vi "DVS_LabVIEWController_april2015.vi"() -> ()   [LabVIEW 2014]
doc: "This example demonstrates temperature control and monitoring.\n\nNote:\nBefore start this VI is it necessary:\n\n- preconfigure some specific parameters that are not supported by this driver (e.g. PV-I/O Type, Linearization type, Alarm Input Values... ) by Quick Codes, or by Eurotherm iTools or by instrument front panel controls\n- enter correct VISA Resource Descriptor, Device Address and Baud Rate into front-panel controls"
uses:
  <vilib>/Instr/_visa.llb/VISA Configure Serial Port (Instr).vi
  Environmental Chamber LabVIEW and Instruments/Drivers and Software/keithley_6430/Keithley 6430/Public/Data/Read (Single Point).vi
  Environmental Chamber LabVIEW and Instruments/Drivers and Software/LabVIEW 8.2 Drivers/keithley_24xx/Keithley 24XX/Public/Data/Read (Single Point).vi
  <vilib>/Utility/file.llb/Write To Spreadsheet File (string).vi
  Environmental Chamber LabVIEW and Instruments/Drivers and Software/keithley_24xx/Keithley 24XX/Keithley 24XX.lvlib
  Environmental Chamber LabVIEW and Instruments/Drivers and Software/keithley_6430/Keithley 6430/Keithley 6430.lvlib
panel:
  out "F_o (MHz)":dbl
  out "Waveform Chart 8":cluster{dbl}(graph)
  out "Waveform Chart 9":cluster{"Measurement":dbl}(graph)
  out "Waveform Chart 4":cluster{"Resistance":sgl}(graph)
  in  "Keithley 6430":bool
  in  "Keithley 2422":bool
  in  "Keithley 2423":bool
  in  "Keithley 2421":bool
  in  "stop":bool
  in  "Keithley 2420":bool
  in  "J-KEM":bool
  out "Start Time":string
  out "Elapsed (min)":dbl caption="Elapsed Time (s)"
  out "Data\nfile\npath":path
  in  "Comments":string
  out "Program Errors":errorcluster
  in  "Delay between data points (s)":dbl min=0.0 max=30.0 format="%#_13g"
  in  "Stop after (min)":dbl
  in  "Auto stop?":bool
  out "Ohm":dbl format="%.4e"
  out "MHz":dbl format="%.6f"
  out "Waveform Chart 7":cluster{dbl, "Resistance out":dbl}(graph)
  out "Waveform Chart 5":cluster{dbl}(graph)
  in  "Clear all charts":bool
  out "Waveform Chart 6":cluster{dbl}(graph)
  out "O2 Concentration (PPM)":dbl
  out "Waveform Chart":cluster{dbl}(graph)
  out "Torr":dbl
  out "%":dbl
  out "atm":dbl
  in  "Com Port":i32(ring) items=["Com 1", "Com 2", "Com 3", "Com 4", "Com 5", "Com 6", "COM 7", "COM 8", "COM 9", "COM 10", "COM 11", "COM 12", "com 13", "COM 14"]
  in  "Baud Rate 2":i32(ring)=2 items=["2400", "4800", "9600", "19200", "38400", "57600", "115200"]
  in  "Com Port 2":i32(ring) items=["Com 1", "Com 2", "Com 3", "Com 4", "Com 5", "Com 6", "COM 7", "COM 8", "COM 9", "COM 10", "COM 11", "COM 12", "com 13", "COM 14"]
  # "Configuring Instrument\n \nPlease Wait......\n\nChart will update in 20 sec"
  # "O2 Partial Pressure"
  # "SetNag\nO2 Pump"
  # "Rapidox O2 Sensor"
  # "°C"
  # "Sample Temperature"
  # "Mass adsorbed (g)"
  # "Keithley 6430 Resistance"
  # "Ohm"
  # "Keithley 2420 Resistance"
  # "Ohm"
  # "Setup"
  # "Instruments Connected:"
  # "Timing"
  # "SRS QCM"
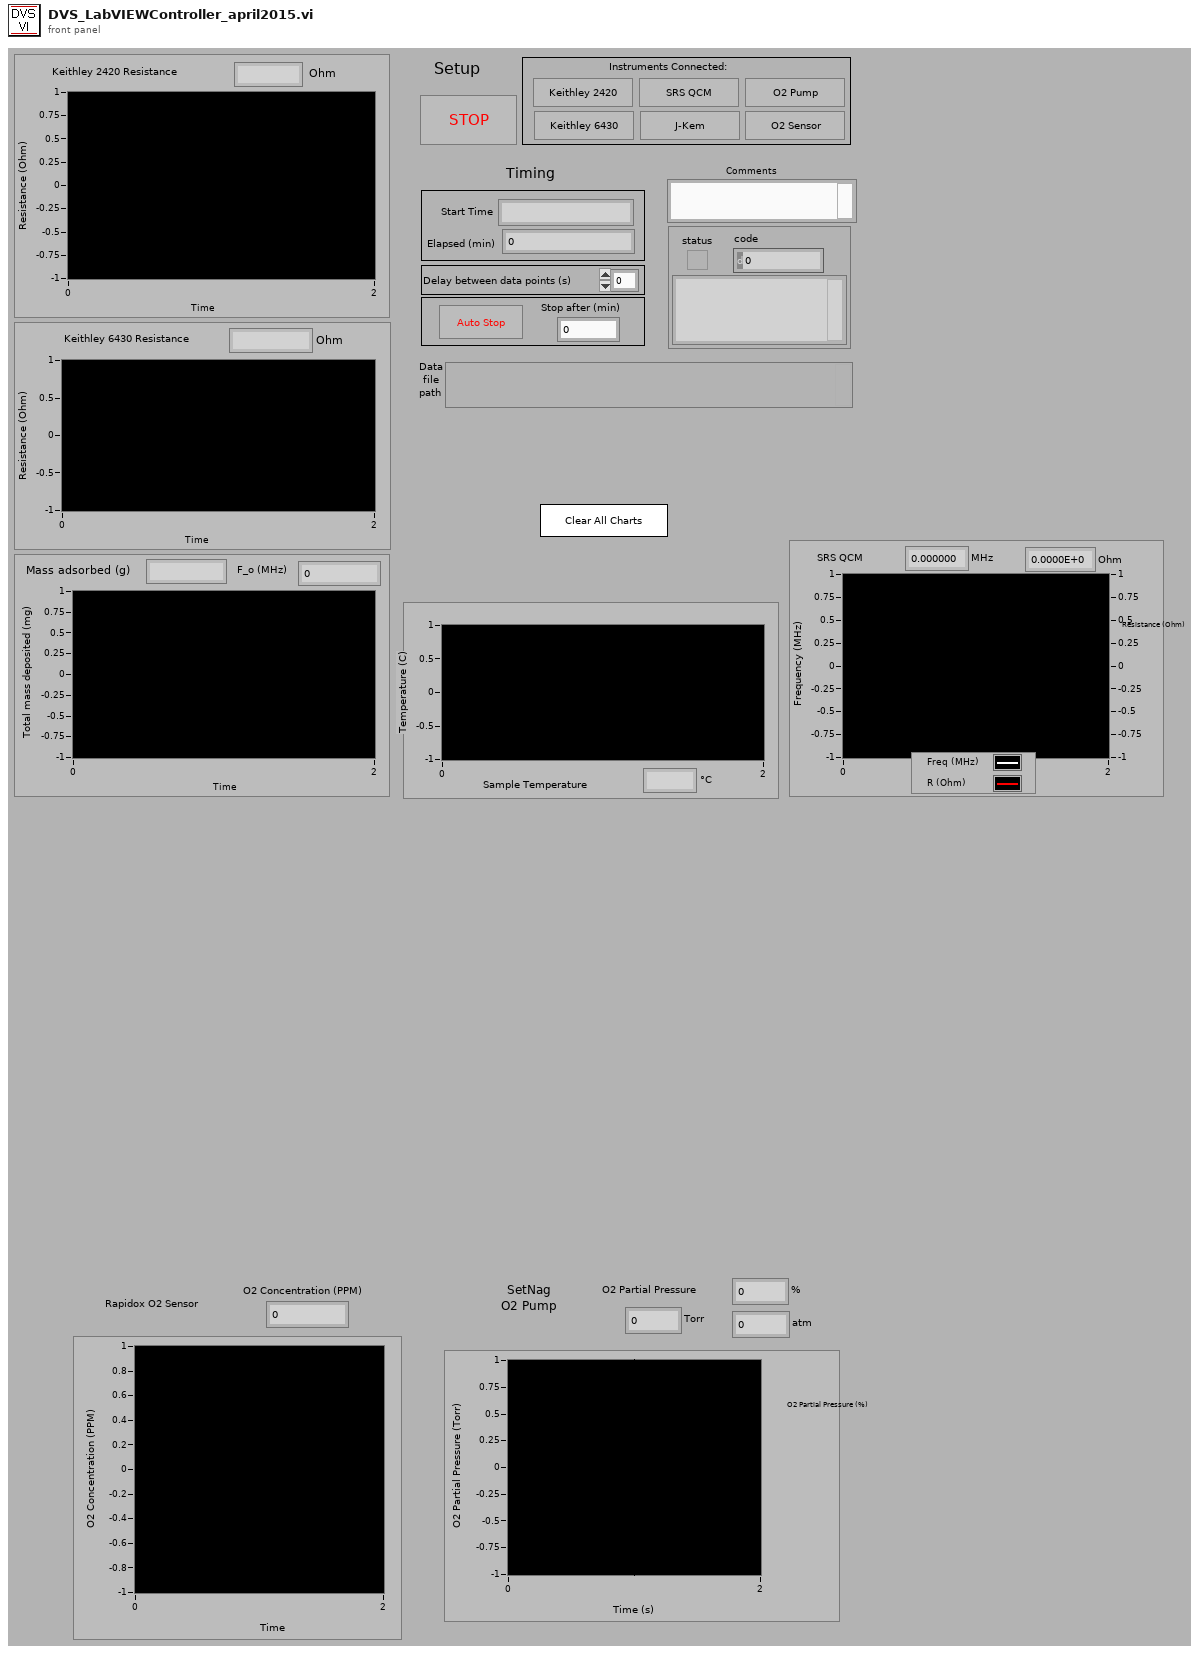
[diagram p1: front panel]
types:
  T1 = enum16{"open", "open or create", "create or replace", "create", "open (read only)"}
  T2 = enum16{"no parity", "odd parity", "even parity", "mark parity", "space parity"}
  T3 = cluster{bool, "VISA resource name":refnum<visa-resource-name>, "error out":errorcluster}
  T4 = cluster{bool, "VISA resource name out":refnum<visa-resource-name>, "error out":errorcluster}
  T5 = cluster{bool, "VISA out":refnum<visa-resource-name>, "error out":errorcluster}
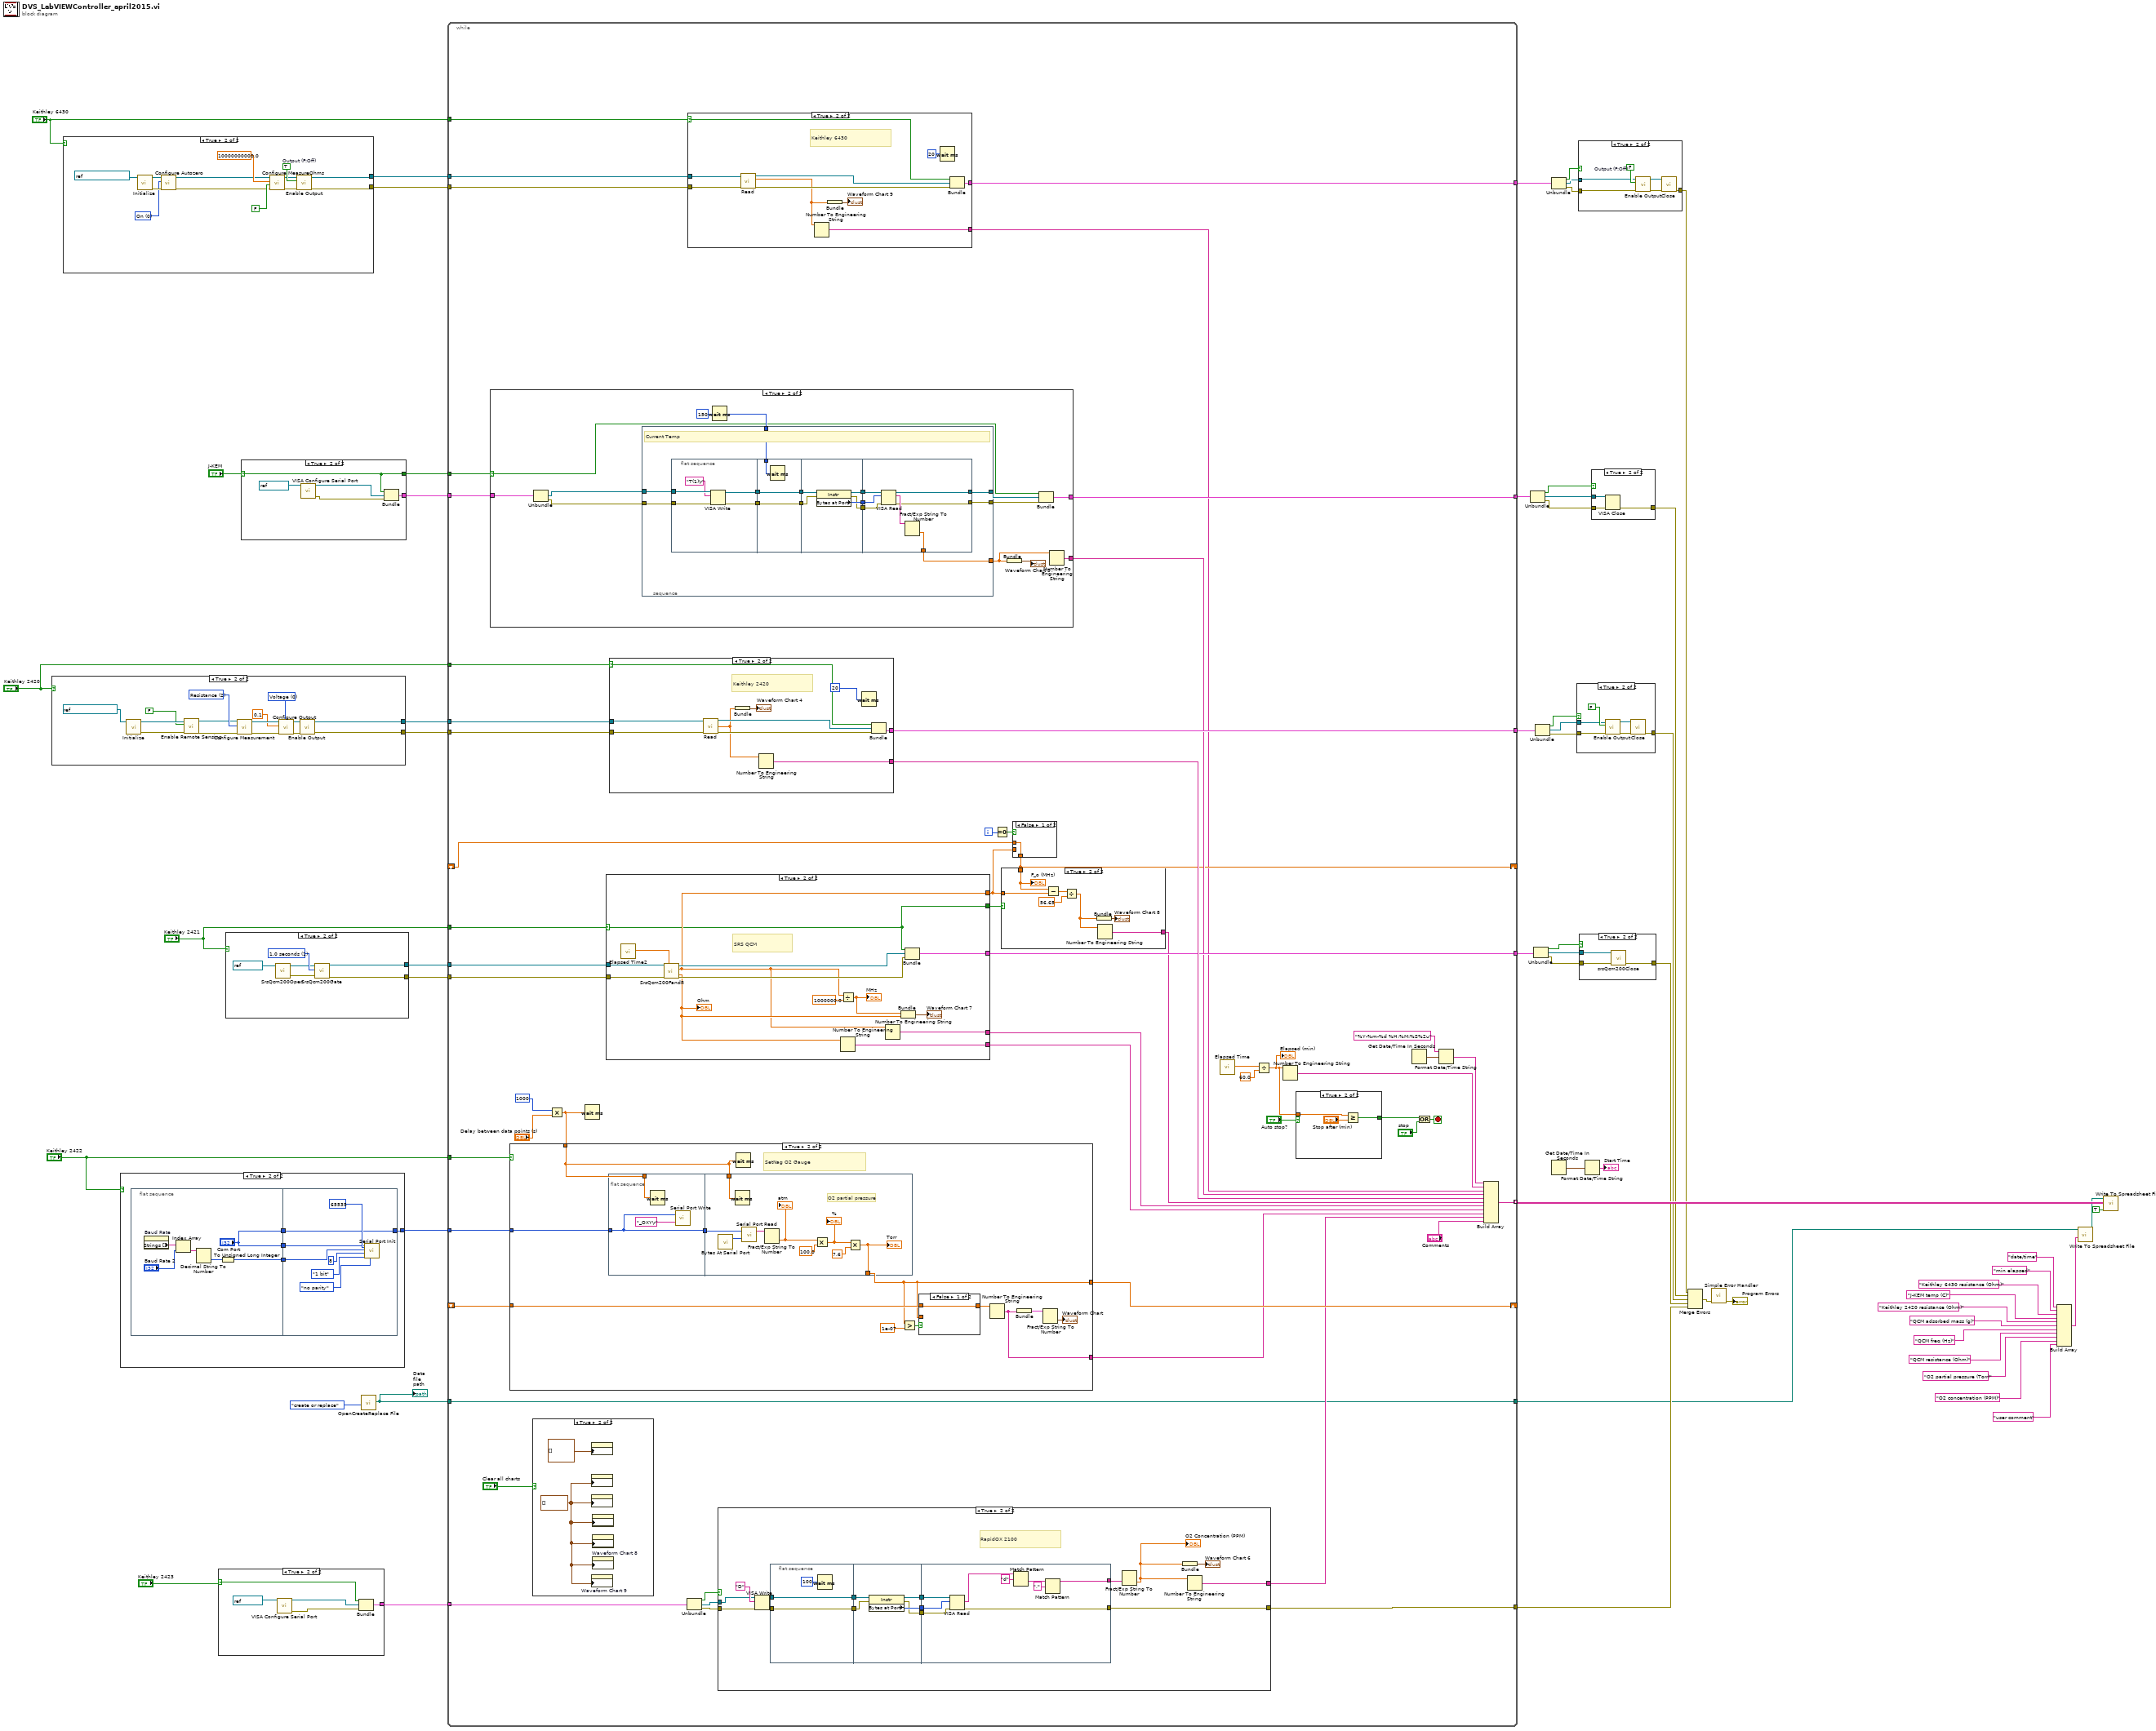
[diagram p0: block diagram]
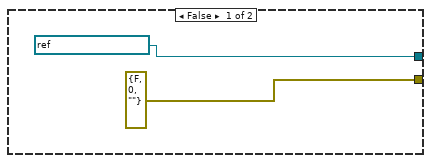
[diagram p3: hidden frame]
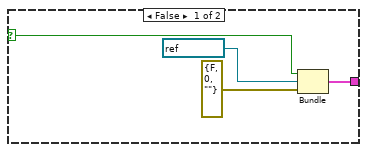
[diagram p4: hidden frame]
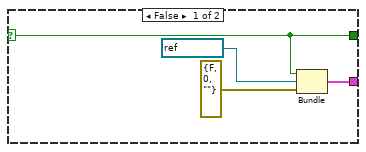
[diagram p6: hidden frame]
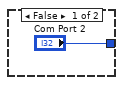
[diagram p7: hidden frame]
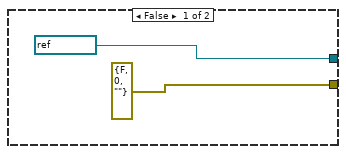
[diagram p9: hidden frame]
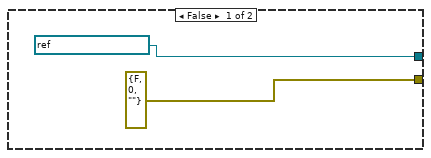
[diagram p11: hidden frame]
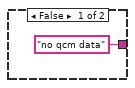
[diagram p12: hidden frame]
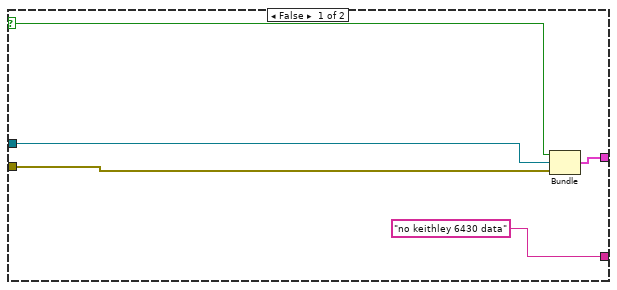
[diagram p13: hidden frame]
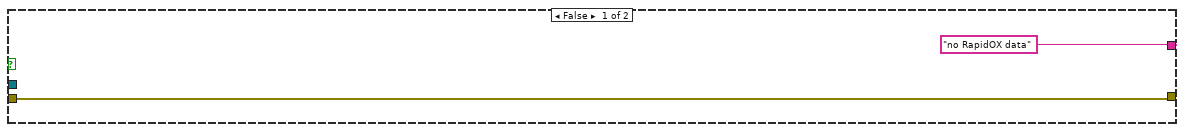
[diagram p16: hidden frame]
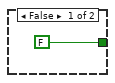
[diagram p17: hidden frame]
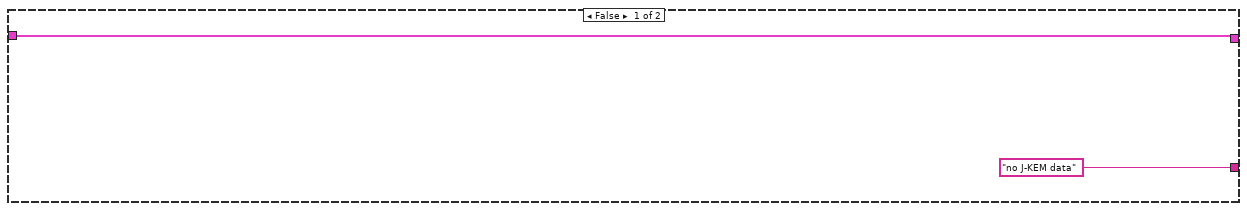
[diagram p18: hidden frame]
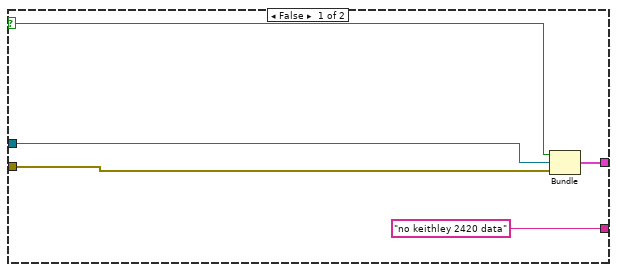
[diagram p19: hidden frame]
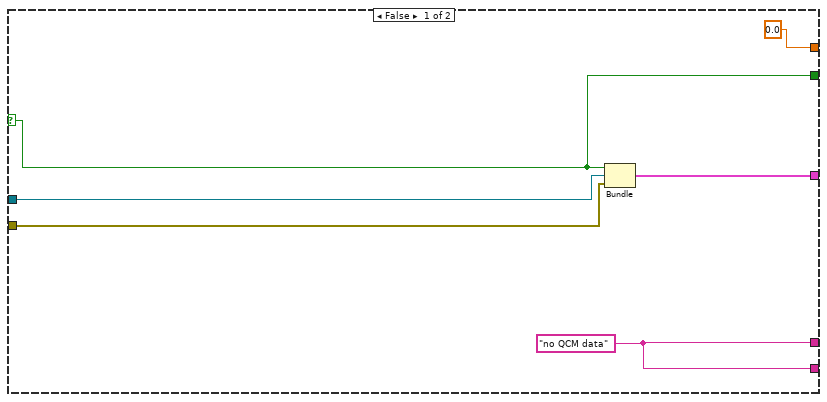
[diagram p20: hidden frame]
diagram:
  n1 = case shown="True" "Keithley 2420" {
    tunnel: [refnum<visa-resource-name> "GPIB1::24::INSTR" ("VISA resource name") w68] -> w54
    tunnel: [errorcluster {"status"=FALSE, "code"=0, "source"=""} ("error out") w63] -> w53
    frame False {
    }
    frame True {
      w70 = u16 0 items=["Voltage", "Current"] ("Source Mode  (0: Voltage)")
      w75 = u16 2 items=["Volts", "Current", "Resistance"] ("Function (0: Volts)")
      n2 = call "Initialize.vi"("VISA resource name"=refnum<visa-resource-name> "GPIB1::24::INSTR") -> ("error out"=w64:errorcluster, "VISA resource name out"=w67:refnum<visa-resource-name>)  [unwired: 9 in]
      n3 = call "Enable Remote Sensing.vi"("error in (no error)"=w64, "Enable Remote Sensing (T: Enable)"=FALSE ("4-wire?"), "VISA resource name"=w67) -> ("error out"=w65:errorcluster, "VISA resource name out"=w66:refnum<visa-resource-name>)  [unwired: 7 in]
      n4 = call "Configure Measurement.vi"("error in (no error)"=w65, "Function (0: Volts)"=w75, "VISA resource name"=w66) -> ("error out"=w74:errorcluster, "VISA resource name out"=w73:refnum<visa-resource-name>)  [unwired: 7 in]
      n5 = call "Configure Output.vi"("Source Mode  (0: Voltage)"=w70, "error in (no error)"=w74, "Output Level (0)"=0.1 ("Applied Voltage (V)"), "VISA resource name"=w73) -> ("error out"=w72:errorcluster, "VISA resource name out"=w71:refnum<visa-resource-name>)  [unwired: 6 in]
      n6 = call "Enable Output.vi"("error in (no error)"=w72, "VISA resource name"=w71) -> ("error out"=w63:errorcluster, "VISA resource name out"=w68:refnum<visa-resource-name>)  [unwired: 8 in]
    }
  }
  n7 = case shown="True" "Keithley 6430" {
    tunnel: [refnum<visa-resource-name> "GPIB0::29::INSTR" ("VISA resource name") w86] -> w6
    tunnel: [errorcluster {"status"=FALSE, "code"=0, "source"=""} ("error out") w87] -> w5
    frame False {
    }
    frame True {
      w82 = u16 0 items=["On", "Off", "Once"] ("Autozero  (0: On)")
      w90 = TRUE  # Output (F:Off)
      n8 = call "Initialize.vi"("VISA resource name"=refnum<visa-resource-name> "GPIB0::29::INSTR") -> ("error out"=w83:errorcluster, "VISA resource name out"=w84:refnum<visa-resource-name>)  [unwired: 4 in, 5 out]
      n9 = call "Configure Autozero.vi"("error in (no error)"=w83, "Autozero  (0: On)"=w82, "VISA resource name"=w84) -> ("error out"=w79:errorcluster, "VISA resource name out"=w80:refnum<visa-resource-name>)  [unwired: 7 in]
      n10 = call "Configure MeasureOhms.vi"("error in (no error)"=w79, "Auto Range (T:Enable)"=FALSE, "Resistance Range [Ohms]"=10000000000.0, "VISA resource name"=w80) -> ("error out"=w91:errorcluster, "VISA resource name out"=w89:refnum<visa-resource-name>)  [unwired: 2 in, 4 out]
      n11 = call "Enable Output.vi"("error in (no error)"=w91, "Enable Output (F:Off)"=w90, "VISA resource name"=w89) -> ("error out"=w87:errorcluster, "VISA resource name out"=w86:refnum<visa-resource-name>)  [unwired: 7 out]
    }
  }
  n12 = case shown="True" "Keithley 2422" {
    tunnel: ["Com Port 2" w93] -> w50
    frame False {
    }
    frame True {
      n13 = flat-sequence {
        tunnel: ["Com Port"] -> w96
        tunnel: [w98] -> w95
        tunnel: ["Com Port"] -> w94
        tunnel: w96 -> [w104]
        tunnel: w95 -> [w103]
        tunnel: w94 -> [w105]
        tunnel: [w105] -> w93
        frame #0 {
          n14 = property on="Baud Rate" class="Ring (strict)"() -> ("Strings []"=w100:string[])  [unwired: 2 in, 2 out]
          n15 = Index Array(array=w100, index="Baud Rate 2") -> (element=w101:string)
          n16 = Decimal String To Number(string=w101) -> (number=w99:i32)  [unwired: 2 in, 1 out]
          n17 = To Unsigned Long Integer(number=w99) -> (unsigned 32bit integer=w98:u32)
        }
        frame #1 {
          n18 = call <vilib>:"Serial Port Init.vi"("parity"=T2."no parity", "buffer size"=u16 65535, "stop bits"=enum16{"1 bit", "1.5 bits", "2 bits"}."1 bit", "data bits"=u16 8, "baud rate"=w103, "port number"=w104) -> ()  [unwired: 1 in, 1 out]
        }
      }
    }
  }
  n19 = case shown="True" "Keithley 2423" {
    selector: "Keithley 2423" -> [w110 w115]
    tunnel: [w111 w116] -> w19
    frame False {
      n20 = Bundle(w110, "VISA resource name"=refnum<visa-resource-name> "COM7", "error out"=errorcluster {"status"=FALSE, "code"=0, "source"=""}) -> (w111:T3)  [unwired: 1 in]
    }
    frame True {
      n21 = call-poly "VISA Configure Serial Port"("VISA resource name"=refnum<visa-resource-name> "COM7") -> ("VISA resource name out"=w117:refnum<visa-resource-name>, "error out"=w114:errorcluster)  [unwired: 13 in]
      n22 = Bundle(w115, "VISA resource name out"=w117, "error out"=w114) -> (w116:T4)  [unwired: 1 in]
    }
  }
  n23 = case shown="True" "Keithley 2421" {
    tunnel: [refnum<visa-resource-name> "COM6" ("VISA in") w122] -> w52
    tunnel: [errorcluster {"status"=FALSE, "code"=0, "source"=""} ("error out") w121] -> w51
    frame False {
    }
    frame True {
      w126 = u16 1 items=["0.1 seconds", "1.0 seconds", "10.0 seconds"] ("Gate in")
      n24 = call "SrsQcm200Open.vi"("VISA in"=refnum<visa-resource-name> "COM6") -> ("error out"=w123:errorcluster, "VISA out"=w124:refnum<visa-resource-name>)  [unwired: 4 in]
      n25 = call "SrsQcm200Gate.vi"("VISA in"=w124, "Gate in"=w126, "error in (no error)"=w123) -> ("VISA out"=w122:refnum<visa-resource-name>, "error out"=w121:errorcluster)  [unwired: 14 in, 1 out]
    }
  }
  n26 = case shown="True" "J-KEM" {
    selector: "J-KEM" -> [w127 w132]
    tunnel: [w128 w133] -> w39
    tunnel: [w127 w132] -> w32
    frame False {
      n27 = Bundle(w127, "VISA resource name"=refnum<visa-resource-name> "COM3", "error out"=errorcluster {"status"=FALSE, "code"=0, "source"=""}) -> (w128:T3)  [unwired: 1 in]
    }
    frame True {
      n28 = call-poly "VISA Configure Serial Port"("VISA resource name"=refnum<visa-resource-name> "COM3") -> ("VISA resource name out"=w134:refnum<visa-resource-name>, "error out"=w131:errorcluster)  [unwired: 13 in]
      n29 = Bundle(w132, "VISA resource name out"=w134, "error out"=w131) -> (w133:T4)  [unwired: 1 in]
    }
  }
  n30 = call "OpenCreateReplace File.vi"("function (open:0)"=T1."create or replace") -> ("new file path"=w15:path)  [unwired: 7 in, 3 out]
  "Data\nfile\npath" <- w15
  n31 = while {
    shift-right: [w189] -> _
    shift-left: _ -> [w188]
    tunnel: [w186] -> w56 mode=indexing
    tunnel: "Keithley 2420" -> [w152]
    tunnel: w54 -> [w184]
    tunnel: w53 -> [w183]
    tunnel: w52 -> [w182]
    tunnel: w51 -> [w181]
    tunnel: "Keithley 2421" -> [w179]
    tunnel: "Keithley 2422" -> [w172]
    tunnel: w50 -> [w178]
    tunnel: [w174] -> w47
    tunnel: [w173] -> w43
    tunnel: w39 -> [w171]
    tunnel: [w170] -> w37
    tunnel: w32 -> [w168]
    tunnel: w19 -> [w161]
    tunnel: [w156] -> w17
    tunnel: [w151] -> w16
    tunnel: w15 -> [w151]
    shift-right: [w145] -> _
    shift-left: _ -> [w144]
    tunnel: w6 -> [w143]
    tunnel: w5 -> [w142]
    tunnel: [w141] -> w3
    tunnel: "Keithley 6430" -> [w140]
    i -> [w137]
    stop <- w166 stop-if-true
    n32 = case shown="True" w168 {
      selector: w168 -> [_ w260]
      tunnel: w171 -> [w258 w265]
      tunnel: [w258 w263] -> w170
      tunnel: ["no J-KEM data" w261] -> w169
      frame False {
      }
      frame True {
        w269 = u32 150 ("milliseconds to wait")
        n33 = Unbundle(w265) -> ("VISA resource name out"=w264:refnum<visa-resource-name>, "error out"=w259:errorcluster)  [unwired: 1 out]
        n34 = stacked-sequence {
          tunnel: w264 -> [w275]
          tunnel: w259 -> [w274]
          tunnel: w269 -> [w273]
          tunnel: [w271] -> w266
          tunnel: [w270] -> w267
          tunnel: [w272] -> w262
          frame #0 {
            # "Current Temp"
            n35 = flat-sequence {
              tunnel: w275 -> [w287]
              tunnel: w274 -> [w286]
              tunnel: [w284] -> w282
              tunnel: [w283] -> w281
              tunnel: w273 -> [w290]
              tunnel: [w289] -> w280
              tunnel: w282 -> [w289]
              tunnel: w281 -> [w288]
              tunnel: [w288] -> w279
              tunnel: w280 -> [w295]
              tunnel: w279 -> [w294]
              tunnel: [w293] -> w278
              tunnel: [w292] -> w277
              tunnel: [w291] -> w276
              tunnel: w278 -> [w302]
              tunnel: w277 -> [w301]
              tunnel: w276 -> [w300]
              tunnel: [w297] -> w270
              tunnel: [w298] -> w271
              tunnel: [w296] -> w272
              frame #0 {
                n36 = VISA Write(VISA resource name=w287, write buffer="T(1)\r", error in (no error)=w286) -> (VISA resource name out=w284:refnum<visa-resource-name>, error out=w283:errorcluster)  [unwired: 1 out]
              }
              frame #1 {
                n37 = Wait (ms)(milliseconds to wait=w290) -> ()  [unwired: 1 out]
              }
              frame #2 {
                n38 = property class="Instr"(reference=w295, error in=w294) -> (reference out=w293:refnum<visa-resource-name>, error out=w291:errorcluster, "Bytes at Port"=w292:u32)
              }
              frame #3 {
                n39 = VISA Read(VISA resource name=w302, byte count=w301, error in (no error)=w300) -> (VISA resource name out=w298:refnum<visa-resource-name>, read buffer=w299:string, error out=w297:errorcluster)  [unwired: 1 out]
                n40 = Fract/Exp String To Number(string=w299) -> (number=w296:dbl)  [unwired: 3 in, 1 out]
              }
            }
          }
        }
        n41 = Wait (ms)(milliseconds to wait=w269) -> ()  [unwired: 1 out]
        n42 = Bundle(w262) -> (→"Waveform Chart 5":cluster{dbl})  [unwired: 1 in]
        n43 = Bundle(w260, "VISA resource name out"=w266, "error out"=w267) -> (w263:T4)  [unwired: 1 in]
        n44 = Number To Engineering String(4:w262) -> (0:w261:string)  [unwired: 3 in]
      }
    }
    n45 = case shown="True" "Clear all charts" {
      frame False {
      }
      frame True {
        w217 = cluster{dbl}[] [] ("History Data")
        n46 = property on="Waveform Chart 7" class="WFChart (strict)"("History Data"=cluster{dbl, "Resistance out":dbl}[] []) -> ()  [unwired: 2 in, 2 out]
        n47 = property on="Waveform Chart 4" class="WFChart (strict)"("History Data"=w217) -> ()  [unwired: 2 in, 2 out]
        n48 = property on="Waveform Chart 5" class="WFChart (strict)"("History Data"=w217) -> ()  [unwired: 2 in, 2 out]
        n49 = property on="Waveform Chart 9" class="WFChart (strict)"("History Data"=w217) -> ()  [unwired: 2 in, 2 out]
        n50 = property on="Waveform Chart" class="WFChart (strict)"("History Data"=w217) -> ()  [unwired: 2 in, 2 out]
        n51 = property on="Waveform Chart 6" class="WFChart (strict)"("History Data"=w217) -> ()  [unwired: 2 in, 2 out]
        n52 = property on="Waveform Chart 8" class="WFChart (strict)"("History Data"=w217) -> ()  [unwired: 2 in, 2 out]
      }
    }
    n53 = Multiply(x=u32 1000, y="Delay between data points (s)") -> (x*y=w155:dbl)
    n54 = case shown="True" w172 {
      tunnel: [w339 w343] -> w189
      tunnel: w188 -> [w339 w344]
      tunnel: w155 -> [_ w340]
      tunnel: w178 -> [_ w342]
      tunnel: ["no GenAir data" w341] -> w177
      frame False {
      }
      frame True {
        # "SetNag O2 Gauge"
        n55 = flat-sequence {
          tunnel: [w353] -> w350
          tunnel: w340 -> [w355]
          tunnel: w342 -> [w353]
          tunnel: w350 -> [w356]
          tunnel: w340 -> [w363]
          tunnel: [w359] -> w343
          frame #0 {
            n56 = Wait (ms)(milliseconds to wait=w355) -> ()  [unwired: 1 out]
            n57 = call <vilib>:"Serial Port Write.vi"("string to write"="_OXY\r" ("O2 partial press"), "port number"=w353) -> ()  [unwired: 1 out]
          }
          frame #1 {
            # "O2 partial pressure"
            n58 = call <vilib>:"Bytes At Serial Port.vi"() -> ("byte count"=w364:u32)  [unwired: 1 in, 1 out]
            n59 = Wait (ms)(milliseconds to wait=w363) -> ()  [unwired: 1 out]
            n60 = call <vilib>:"Serial Port Read.vi"("requested byte count"=w364, "port number"=w356) -> ("string read"=w362:string)  [unwired: 1 out]
            n61 = Fract/Exp String To Number(string=w362) -> (number=w360:dbl)  [unwired: 3 in, 1 out]
            "atm" <- w360
            n62 = Multiply(x=w360, y=100.0) -> (x*y=w357:dbl)
            "%" <- w357
            n63 = Multiply(x=w357, y=7.6) -> (x*y=w359:dbl)
            "Torr" <- w359
          }
        }
        n64 = Wait (ms)(milliseconds to wait=w340) -> ()  [unwired: 1 out]
        n65 = Greater?(x=w343, y=1e-07) -> (0:w346:bool)
        n66 = case shown="False" w346 {
          tunnel: [w351 w352] -> w345
          tunnel: w343 -> [_ w352]
          tunnel: w344 -> [w351 _]
          frame False {
          }
          frame True {
          }
        }
        n67 = Number To Engineering String(4:w345) -> (0:w341:string)  [unwired: 3 in]
        n68 = Bundle(w341) -> (w348:cluster{string})  [unwired: 1 in]
        n69 = Fract/Exp String To Number(string=w348) -> (number=→"Waveform Chart":cluster{dbl})  [unwired: 3 in, 1 out]
      }
    }
    n70 = Wait (ms)(milliseconds to wait=w155) -> ()  [unwired: 1 out]
    n71 = case shown="True" w179 {
      selector: w179 -> [w318 w324]
      tunnel: w182 -> [w322 w330]
      tunnel: w181 -> [w321 w332]
      tunnel: [w323 w337] -> w180
      tunnel: [w323 w336] -> w176
      tunnel: [w320 w335] -> w173
      tunnel: [0.0 w325] -> w147
      tunnel: [w318 w324] -> w136
      frame False {
        w323 = "no QCM data"
        n72 = Bundle(w318, "VISA out"=w322, "error out"=w321) -> (w320:T5)  [unwired: 1 in]
      }
      frame True {
        # "SRS QCM"
        n73 = call "Elapsed Time2"() -> ("Elapsed Time (s)"=w331:dbl)  [unwired: 12 in, 7 out]
        n74 = call "SrsQcm200FandR.vi"("VISA in"=w330, "Reference time in"=w331, "error in (no error)"=w332) -> ("VISA out"=w328:refnum<visa-resource-name>, "Frequency out"=w325:dbl, "Resistance out"=w327:dbl, "error out"=w329:errorcluster)  [unwired: 6 in, 3 out]
        "Ohm" <- w327
        n75 = Number To Engineering String(4:w327) -> (0:w336:string)  [unwired: 3 in]
        n76 = Divide(x=w325, y=1000000.0) -> (x/y=w326:dbl)
        "MHz" <- w326
        n77 = Number To Engineering String(4:w325) -> (0:w337:string)  [unwired: 3 in]
        n78 = Bundle(w326, "Resistance out"=w327) -> (→"Waveform Chart 7":cluster{dbl, "Resistance out":dbl})  [unwired: 1 in]
        n79 = Bundle(w324, "VISA out"=w328, "error out"=w329) -> (w335:T5)  [unwired: 1 in]
      }
    }
    n80 = case shown="True" w152 {
      selector: w152 -> [w306 w314]
      tunnel: w184 -> [w305 w309]
      tunnel: w183 -> [w304 w308]
      tunnel: [w303 w312] -> w174
      tunnel: ["no keithley 2420 data" w311] -> w175
      frame False {
        n81 = Bundle(w306, "VISA resource name out"=w305, "error out"=w304) -> (w303:T4)  [unwired: 1 in]
      }
      frame True {
        # "Keithley 2420"
        n82 = call-poly "Read.vi"("VISA resource name"=w309, "error in (no error)"=w308) -> ("VISA resource name out"=w315:refnum<visa-resource-name>, "Resistance"=w310:sgl, "error out"=w313:errorcluster)  [unwired: 7 in, 4 out]
        n83 = Bundle("Resistance"=w310) -> (→"Waveform Chart 4":cluster{"Resistance":sgl})  [unwired: 1 in]
        n84 = Number To Engineering String(4:w310) -> (0:w311:string)  [unwired: 3 in]
        n85 = Wait (ms)(milliseconds to wait=u32 20) -> ()  [unwired: 1 out]
        n86 = Bundle(w314, "VISA resource name out"=w315, "error out"=w313) -> (w312:T4)  [unwired: 1 in]
      }
    }
    n87 = Unbundle(w161) -> (w160:bool, "VISA resource name out"=w159:refnum<visa-resource-name>, "error out"=w158:errorcluster)
    n88 = case shown="True" w140 {
      selector: w140 -> [w203 w213]
      tunnel: w143 -> [w202 w210]
      tunnel: w142 -> [w201 w209]
      tunnel: ["no keithley 6430 data" w212] -> w139
      tunnel: [w200 w211] -> w141
      frame False {
        n89 = Bundle(w203, "VISA resource name out"=w202, "error out"=w201) -> (w200:T4)  [unwired: 1 in]
      }
      frame True {
        # "Keithley 6430"
        n90 = call-poly "Read.vi"("error in (no error)"=w209, "VISA resource name"=w210) -> ("error out"=w208:errorcluster, "Measurement"=w206:dbl, "VISA resource name out"=w207:refnum<visa-resource-name>)  [unwired: 1 in, 6 out]
        n91 = Number To Engineering String(4:w206) -> (0:w212:string)  [unwired: 3 in]
        n92 = Bundle("Measurement"=w206) -> (→"Waveform Chart 9":cluster{"Measurement":dbl})  [unwired: 1 in]
        n93 = Wait (ms)(milliseconds to wait=u32 20) -> ()  [unwired: 1 out]
        n94 = Bundle(w213, "VISA resource name out"=w207, "error out"=w208) -> (w211:T4)  [unwired: 1 in]
      }
    }
    n95 = case shown="True" w160 {
      tunnel: w159 -> [_ w226]
      tunnel: w158 -> [w219 w225]
      tunnel: ["no RapidOX data" w224] -> w157
      tunnel: [w219 w221] -> w156
      frame False {
      }
      frame True {
        # "RapidOX 2100"
        n96 = VISA Write(VISA resource name=w226, write buffer="D", error in (no error)=w225) -> (VISA resource name out=w229:refnum<visa-resource-name>, error out=w228:errorcluster)  [unwired: 1 out]
        n97 = flat-sequence {
          tunnel: [w238] -> w235
          tunnel: [w236] -> w234
          tunnel: w229 -> [w238]
          tunnel: w228 -> [w236]
          tunnel: w235 -> [w243]
          tunnel: w234 -> [w242]
          tunnel: [w241] -> w233
          tunnel: [w240] -> w232
          tunnel: [w239] -> w231
          tunnel: w233 -> [w252]
          tunnel: w232 -> [w251]
          tunnel: w231 -> [w250]
          tunnel: [w249] -> w221
          tunnel: [w244] -> w223
          frame #0 {
            n98 = Wait (ms)(milliseconds to wait=u32 100) -> ()  [unwired: 1 out]
          }
          frame #1 {
            n99 = property class="Instr"(reference=w243, error in=w242) -> (reference out=w241:refnum<visa-resource-name>, error out=w239:errorcluster, "Bytes at Port"=w240:u32)
          }
          frame #2 {
            n100 = VISA Read(VISA resource name=w252, byte count=w251, error in (no error)=w250) -> (read buffer=w247:string, error out=w249:errorcluster)  [unwired: 2 out]
            n101 = Match Pattern(string=w247, regular expression="d") -> (after substring=w245:string)  [unwired: 1 in, 3 out]
            n102 = Match Pattern(string=w245, regular expression=",") -> (before substring=w244:string)  [unwired: 1 in, 3 out]
          }
        }
        n103 = Fract/Exp String To Number(string=w223) -> (number=w222:dbl)  [unwired: 3 in, 1 out]
        "O2 Concentration (PPM)" <- w222
        n104 = Bundle(w222) -> (→"Waveform Chart 6":cluster{dbl})  [unwired: 1 in]
        n105 = Number To Engineering String(4:w222) -> (0:w224:string)  [unwired: 3 in]
      }
    }
    n106 = Equal To 0?(x=w137) -> (x = 0?=w148:bool)
    n107 = case shown="False" w148 {
      tunnel: w147 -> [_ w216]
      tunnel: [w215 w216] -> w145
      tunnel: w144 -> [w215 _]
      frame False {
      }
      frame True {
      }
    }
    n108 = case shown="True" w136 {
      tunnel: w147 -> [_ w197]
      tunnel: ["no qcm data" w195] -> w146
      tunnel: w145 -> [_ w194]
      frame False {
      }
      frame True {
        n109 = Subtract(x=w194, y=w197) -> (x-y=w198:dbl)
        n110 = Divide(x=w198, y=56.65) -> (x/y=w193:dbl)
        n111 = Bundle(w193) -> (→"Waveform Chart 8":cluster{dbl})  [unwired: 1 in]
        n112 = Number To Engineering String(4:w193) -> (0:w195:string)  [unwired: 3 in]
        "F_o (MHz)" <- w194
      }
    }
    n113 = call "Elapsed Time"() -> ("Elapsed Time (s)"=w165:dbl)  [unwired: 12 in, 7 out]
    n114 = Divide(x=w165, y=60.0) -> (x/y=w149:dbl)
    "Elapsed (min)" <- w149
    n115 = Number To Engineering String(4:w149) -> (0:w190:string)  [unwired: 3 in]
    n116 = case shown="True" "Auto stop?" {
      tunnel: [FALSE w256] -> w162
      tunnel: w149 -> [_ w254]
      frame False {
      }
      frame True {
        n117 = Greater Or Equal?(x=w254, y="Stop after (min)") -> (x >= y?=w256:bool)
      }
    }
    n118 = Get Date/Time In Seconds() -> (seconds since 1Jan1904=w191:timestamp)
    n119 = Or(x=w162, y="stop") -> (x .or. y?=w166:bool)
    n120 = Format Date/Time String(time format string (%c)="%Y-%m-%d %H:%M:%S%2u", seconds (now)=w191) -> (date/time string=w185:string)  [unwired: 1 in]
    n121 = Build Array(w185, w190, w139, w169, w175, w146, w180, w176, w177, w157, "Comments") -> (w186:string[])
  }
  n122 = Unbundle(w37) -> (w36:bool, "VISA resource name out"=w35:refnum<visa-resource-name>, "error out"=w34:errorcluster)
  n123 = Unbundle(w43) -> (w42:bool, "VISA out"=w41:refnum<visa-resource-name>, "error out"=w40:errorcluster)
  n124 = Unbundle(w47) -> (w46:bool, "VISA resource name out"=w45:refnum<visa-resource-name>, "error out"=w44:errorcluster)
  n125 = Unbundle(w3) -> (w9:bool, "VISA resource name out"=w8:refnum<visa-resource-name>, "error out"=w7:errorcluster)
  n126 = Get Date/Time In Seconds() -> (seconds since 1Jan1904=w58:timestamp)
  n127 = case shown="True" w46 {
    tunnel: w45 -> [_ w368]
    tunnel: w44 -> [w365 w367]
    tunnel: [w365 w366] -> w48
    frame False {
    }
    frame True {
      n128 = call "Enable Output.vi"("error in (no error)"=w367, "Enable Output (T: Enable)"=FALSE, "VISA resource name"=w368) -> ("error out"=w369:errorcluster, "VISA resource name out"=w371:refnum<visa-resource-name>)  [unwired: 7 in]
      n129 = call "Close.vi"("error in (no error)"=w369, "VISA resource name"=w371) -> ("error out"=w366:errorcluster)  [unwired: 9 in]
    }
  }
  n130 = case shown="True" w9 {
    tunnel: w8 -> [_ w374]
    tunnel: w7 -> [w372 w373]
    tunnel: [w372 w375] -> w2
    frame False {
    }
    frame True {
      w378 = FALSE  # Output (F:Off)
      n131 = call "Enable Output.vi"("error in (no error)"=w373, "Enable Output (F:Off)"=w378, "VISA resource name"=w374) -> ("error out"=w376:errorcluster, "VISA resource name out"=w377:refnum<visa-resource-name>)  [unwired: 7 out]
      n132 = call "Close.vi"("error in (no error)"=w376, "VISA resource name"=w377) -> ("error out"=w375:errorcluster)  [unwired: 9 out]
    }
  }
  n133 = case shown="True" w42 {
    tunnel: w40 -> [w379 w382]
    tunnel: [w379 w381] -> w49
    tunnel: w41 -> [_ w380]
    frame False {
    }
    frame True {
      n134 = call "srsQcm200Close.vi"("error in"=w382, "Visa in"=w380) -> ("error out"=w381:errorcluster)  [unwired: 3 in]
    }
  }
  n135 = Format Date/Time String(seconds (now)=w58) -> (date/time string=→"Start Time":string)  [unwired: 2 in]
  n136 = case shown="True" w36 {
    tunnel: w35 -> [_ w386]
    tunnel: w34 -> [w383 w385]
    tunnel: [w383 w384] -> w33
    frame False {
    }
    frame True {
      n137 = VISA Close(VISA resource name=w386, error in (no error)=w385) -> (error out=w384:errorcluster)
    }
  }
  n138 = Merge Errors(w2, w33, w48, w49, w17) -> (w57:errorcluster)
  n139 = call <vilib>:"Simple Error Handler.vi"("error in (no error)"=w57) -> ("error out"=→"Program Errors":errorcluster)  [unwired: 4 in, 4 out]
  n140 = Build Array("date/time", "min elapsed", "Keithley 6430 resistance (Ohm)", "J-KEM temp (C)", "Keithley 2420 resistance (Ohm)" ("element"), "QCM adsorbed mass (g)", "QCM freq (Hz)", "QCM resistance (Ohm)", "O2 partial pressure (Torr)" ("element"), "O2 concentration (PPM)" ("element"), "user comment" ("element")) -> (w24:string[])
  n141 = call-poly <vilib>:"Write To Spreadsheet File.vi"("1D data"=w24, "file path (dialog if empty)"=w16) -> ("new file path (Not A Path if cancelled)"=w25:path)  [unwired: 6 in]
  n142 = call-poly <vilib>:"Write To Spreadsheet File.vi"("append to file? (new file:F)"=TRUE, "2D data"=w56, "file path (dialog if empty)"=w25) -> ()  [unwired: 5 in, 1 out]
